vi "Assertion Failure Message.vi"() -> ()   [LabVIEW 2017, in "Transparent Assertions.Tests.lvlib" / "Assert Not Equal.lvlib"]
uses:
  Assert Not Equal.lvlib
  src/Transparent Assertions/Transparent Assertions.lvlib
panel:
  out "error out":errorcluster
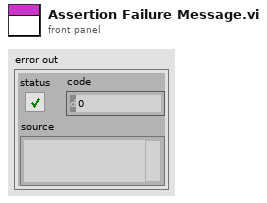
[diagram p1: front panel]
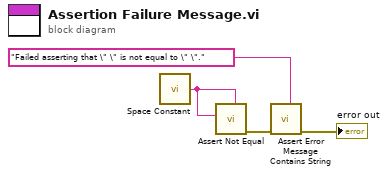
[diagram p0: block diagram]
diagram:
  n1 = call <vilib>:"Space Constant.vi"() -> ("String"=w1:string)
  n2 = call "Assert Not Equal.vi"("Expected"=w1, "Actual"=w1) -> ("error out"=w4:errorcluster)  [unwired: 9 in]
  n3 = call "Assert Error Message Contains String.vi"("Expected"="Failed asserting that \" \" is not equal to \" \"." ("y"), "error in (no error)"=w4) -> ("error out"=→"error out":errorcluster)  [unwired: 9 in]
